vi "Read Digital Input Module.vi"   [LabVIEW 2017, in "Scan Engine Scripting.lvlib"]
uses:
  Scan Engine Scripting.lvlib
  NI 9422/NI 9422.lvclass
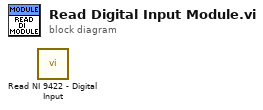
[diagram p0: block diagram]
diagram:
  n1 = call "Read NI 9422 - Digital Input.vi"() -> ()  [unwired: 9 in, 3 out]
